vi "gfitsio-movnam-hdu.vi"(7 "extname":string, 8 "error in (no error)":errorcluster, 9 "extver (0:ignore extver)":i32, 10 "hdutype (ANY_HDU)":T2=-1 items=["ANY_HDU"=-1, "IMAGE_HDU"=0, "ASCII_TBL"=1, "BINARY_TBL"=2], 11 "gfits refnum":T1) -> (0 "error out":errorcluster, 3 "dup gfits refnum":T1)   [LabVIEW 2023, in "gfitsio.lvlib"]
doc: "Moves to the (first) HDU which has the specified extension type and EXTNAME and EXTVER keyword values (or HDUNAME and HDUVER keywords). The hdutype parameter may have a value of IMAGE_HDU, ASCII_TBL, BINARY_TBL, or ANY_HDU where ANY_HDU means that only the extname and extver values will be used to locate the correct extension. If the input value of extver is 0 then the EXTVER keyword is ignored and the first HDU with a matching EXTNAME (or HDUNAME) keyword will be found. If no matching HDU is found in the file then the current HDU will remain unchanged and an error will be returned."
uses:
  gfitsio.lvlib
  gfitsio.dll
  gfitsio-refnum.ctl
  cfitsio-hdutypes.ctl
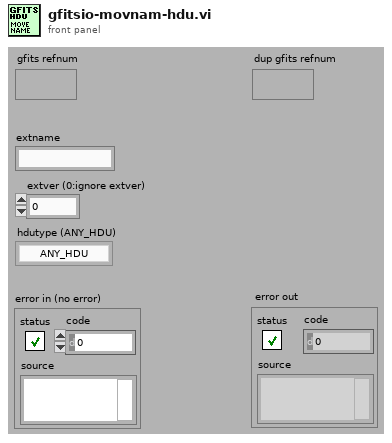
[diagram p1: front panel]
types:
  T1 = typedef "gfitsio.lvlib/gfitsio-refnum.ctl" = refnum<k1>
  T2 = typedef "gfitsio.lvlib/cfitsio-hdutypes.ctl" = i32
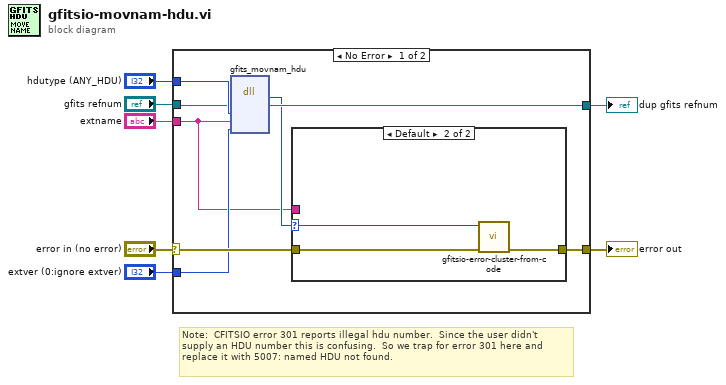
[diagram p0: block diagram]
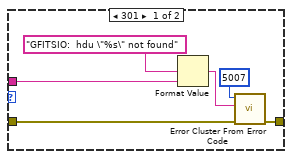
[diagram p2: hidden frame]
diagram:
  # "Note:  CFITSIO error 301 reports illegal hdu number.  Since the user didn't supply an HDU number this is confusing.  So we trap for error 301 here and replace it with 5007: named HDU not found."
  n1 = case shown="No Error" "error in (no error)" {
    selector: "error in (no error)" -> [w15 w26]
    tunnel: [w14 w26] -> w6
    tunnel: "extname" -> [w8 _]
    tunnel: "extver (0:ignore extver)" -> [w13 _]
    tunnel: "hdutype (ANY_HDU)" -> [w12 _]
    tunnel: [w10 w25] -> w2
    tunnel: "gfits refnum" -> [w11 w25]
    frame No Error {
      n2 = dll-call lib="gfitsio.dll" fn="gfits_movnam_hdu"("refnum"=w11, "hdutype"=w12, "extname"=w8, "extver"=w13) -> (w9:i32, "refnum"=w10:T1)  [unwired: 5 in, 3 out]
      n3 = case shown="Default" w9 {
        selector: w9 -> [_ w22]
        tunnel: w15 -> [w20 w24]
        tunnel: [w21 w23] -> w14
        tunnel: w8 -> [w17 _]
        frame 301 {
          n4 = Format Value(format string="GFITSIO:  hdu \"%s\" not found", value (0)=w17) -> (output string=w19:string)  [unwired: 1 out]
          n5 = call <vilib>:"Error Cluster From Error Code.vi"("error in (no error)"=w20, "error message (\"\")"=w19, "error code (0)"=5007) -> ("error out"=w21:errorcluster)  [unwired: 1 in, 5 out]
        }
        frame Default {
          n6 = call "gfitsio-error-cluster-from-code.vi"("error in (no error)"=w24, "error code"=w22) -> ("error out"=w23:errorcluster)  [unwired: 9 out]
        }
      }
    }
    frame Error {
    }
  }
  "error out" <- w6
  "dup gfits refnum" <- w2
